vi "FT10_Read Stop Notifier.vi"(8 "error in (no error)":errorcluster) -> (0 "error out":errorcluster, 3 "Stop Notifier":bool)   [LabVIEW 2015]
doc: "Gets status from stop notifier."
uses:
  Controls/Config_Stop Notifier Enum.ctl
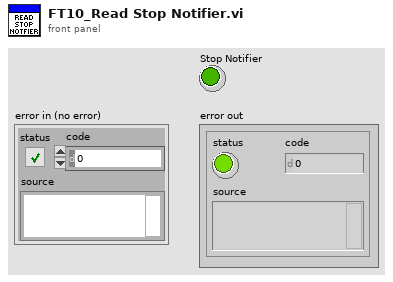
[diagram p1: front panel]
types:
  T1 = typedef "Config_Stop Notifier Enum.ctl" = enum16{"Initialize", "Read Notifier", "Notify", "Close"}
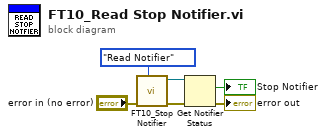
[diagram p0: block diagram]
diagram:
  n1 = call "FT10_Stop Notifier.vi"("Selector"=Config_Stop_Notifier_Enum."Read Notifier", "error in (no error)"="error in (no error)") -> ("error out"=w3:errorcluster, "Notifier out"=w2:refnum<notifier>)  [unwired: 8 in]
  n2 = Get Notifier Status(notifier=w2, error in (no error)=w3) -> (current notification=→"Stop Notifier":bool, error out=→"error out":errorcluster)  [unwired: 3 out]
